vi "Temp Property Node_Remove.vi"(8 "error in":errorcluster, 11 "Temp Ref Out":refnum<vi>) -> (0 "error out":errorcluster)   [LabVIEW 2023]
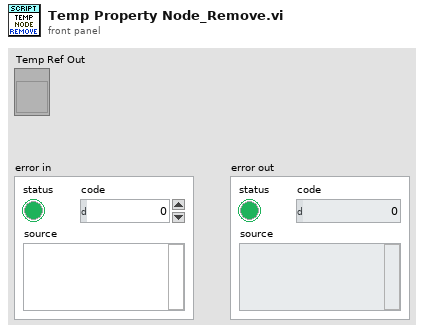
[diagram p1: front panel]
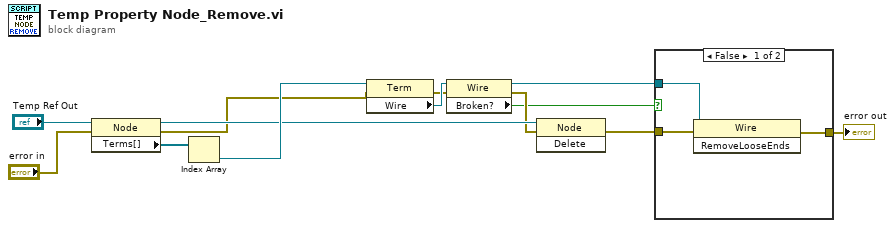
[diagram p0: block diagram]
diagram:
  n1 = property class="Node"(reference="Temp Ref Out", error in="error in") -> (reference out=w8:refnum<vi>, error out=w7:errorcluster, "Terms[]"=w10:refnum<vi>[])
  n2 = Index Array(array=w10) -> (element=w9:refnum<vi>)  [unwired: 1 in]
  n3 = property class="Term"(reference=w9, error in=w7) -> (error out=w12:errorcluster, "Wire"=w13:refnum<vi>)  [unwired: 1 out]
  n4 = property class="Wire"(reference=w13, error in=w12) -> (reference out=w1:refnum<vi>, error out=w6:errorcluster, "Broken?"=w4:bool)
  n5 = invoke class="Node" method="Delete"(reference=w8, error in=w6) -> (error out=w5:errorcluster)  [unwired: 1 in, 2 out]
  n6 = case shown="False" w4 {
    tunnel: [w16 w17] -> w2
    tunnel: w5 -> [w15 w17]
    tunnel: w1 -> [w14 _]
    frame False {
      n7 = invoke class="Wire" method="RemoveLooseEnds"(reference=w14, error in=w15) -> (error out=w16:errorcluster)  [unwired: 1 in, 2 out]
    }
    frame True {
    }
  }
  "error out" <- w2
